vi "Flush.vi"(8 "error in (no error)":errorcluster, 9 "Single / Multivalve?":bool, 10 "Channel":u32, 11 "LINX Resource":T1={"IO"=enum."Remote", "Interface"=enum."Serial", "LINX Device Config"={"Interface"=enum."Serial", "COM Port"="COM13", "TCP Configuration"={"IP Address"="", "Port"=0}, "Device Family"=1, "Device ID"=1, "Device Name"="myRIO-1900", "TCP Ref"=refnum, "Channels"={"DI"=[0, 1, 2, 3, 4, 5, 6, 7, 8, 9, 10, 11, 12, 13, 14, 15, 16, 17, 18, 19, 20, 21, 22, 23, 24, 25, 26, 27, 28, 29, 30, 31, 32, 33, 34, 35, 36, 37, 38, 39, 40, 41, 42, 43, 44, 45, 46], "DO"=[0, 1, 2, 3, 4, 5, 6, 7, 8, 9, 10, 11, 12, 13, 14, 15, 16, 17, 18, 19, 20, 21, 22, 23, 24, 25, 26, 27, 28, 29, 30, 31, 32, 33, 34, 35, 36, 37, 38, 39, 40, 41, 42, 43, 44, 45, 46], "AI"=[0, 1, 2, 3, 4, 5, 6, 7, 8, 9, 10, 11], "AO"=[], "PWM"=[3, 5, 6, 9, 10], "QE"=[], "UART"=[0, 1], "I2C 2"=[0], "SPI"=[0], "CAN"=[], "Servo"=[], "AI Ref (V)"=0.0, "AI Resolution (Bits)"=0, "AO Ref (V)"=0.0, "AO Resolution (Bits)"=0}}}) -> (0 "error out":errorcluster, 3 "LINX Resource out":T1)   [LabVIEW 2018]
uses:
  <vilib>/MakerHub/LINX/Private/Type Defs/LINX Ref.ctl
  <vilib>/MakerHub/LINX/Private/Type Defs/Platform.ctl
  <vilib>/MakerHub/LINX/Private/Type Defs/Interface.ctl
  <vilib>/MakerHub/LINX/Private/Device/Type Defs/LINX Device Config.ctl
  <vilib>/MakerHub/LINX/Private/Device/Type Defs/TCP Config.ctl
  <vilib>/MakerHub/LINX/Private/Device/Type Defs/Channels.ctl
  <vilib>/MakerHub/LINX/Public/Peripherals/Digital/Digital Write N Chans.vi
  <vilib>/MakerHub/LINX/Private/Local IO/LinxDigitalWrite.vi
  <vilib>/MakerHub/LINX/Public/Utilities/Check Channel.vi
  <vilib>/MakerHub/LINX/Private/Utilties/Generate Error.vi
  <vilib>/MakerHub/LINX/LMH-LINX.lvlib
  <vilib>/MakerHub/LINX/Private/Device/Device.lvlib
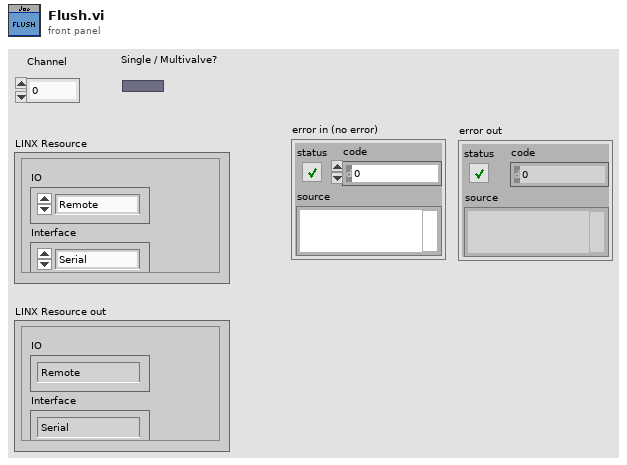
[diagram p1: front panel]
types:
  T1 = typedef "LMH-LINX.lvlib/LINX Ref.ctl" = cluster{"IO":T2, "Interface":T3, "LINX Device Config":T4}
  T2 = typedef "LMH-LINX.lvlib/Platform.ctl" = enum16{"Remote", "Local"}
  T3 = typedef "LMH-LINX.lvlib/Interface.ctl" = enum16{"Serial", "TCP"}
  T4 = typedef "LMH-LINX.lvlib/Device.lvlib/LINX Device Config.ctl" = cluster{"Interface":T3, "COM Port":refnum<visa-resource-name>, "TCP Configuration":T5, "Device Family":u8, "Device ID":u8, "Device Name":string, "TCP Ref":refnum<k5>, "Channels":T6}
  T5 = typedef "LMH-LINX.lvlib/Device.lvlib/TCP Config.ctl" = cluster{"IP Address":string, "Port":u16}
  T6 = typedef "LMH-LINX.lvlib/Channels.ctl" = cluster{"DI":u8[], "DO":u8[], "AI":u8[], "AO":u8[], "PWM":u8[], "QE":u8[], "UART":u8[], "I2C 2":u8[], "SPI":u8[], "CAN":u8[], "Servo":u8[], "AI Ref (V)":dbl, "AI Resolution (Bits)":u8, "AO Ref (V)":dbl, "AO Resolution (Bits)":u8}
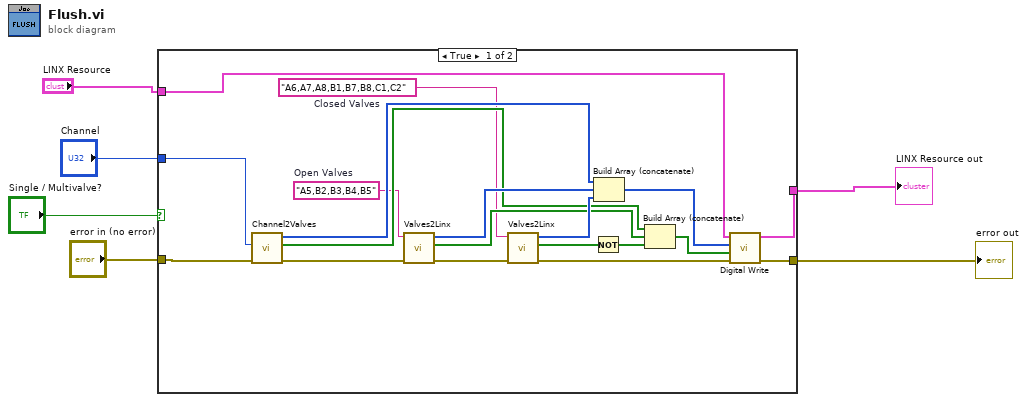
[diagram p0: block diagram]
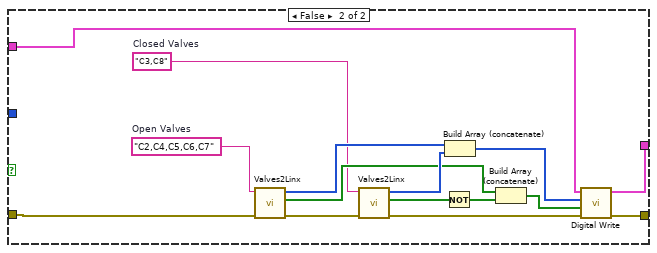
[diagram p2: hidden frame]
diagram:
  n1 = case shown="True" "Single / Multivalve?" {
    tunnel: "error in (no error)" -> [w25 w26]
    tunnel: [w24 w40] -> w5
    tunnel: [w23 w39] -> w4
    tunnel: "Channel" -> [w8 _]
    tunnel: "LINX Resource" -> [w7 w27]
    frame True {
      w9 = "A6,A7,A8,B1,B7,B8,C1,C2"  # Closed Valves
      w10 = "A5,B2,B3,B4,B5"  # Open Valves
      n2 = call "Channel2Valves.vi"("Channel"=w8, "error in (no error)"=w25) -> ("Valve Nums"=w15:i32[], "Valve State"=w14:bool[], "error out"=w13:errorcluster)  [unwired: 6 in]
      n3 = call "Valves2Linx.vi"("error in (no error)"=w13, "Valve (A1-C8),\n comma separated"=w10) -> ("error out"=w17:errorcluster, "Array"=w19:bool[], "Array 2"=w20:i32[])  [unwired: 7 in]
      n4 = call "Valves2Linx.vi"("error in (no error)"=w17, "Valve (A1-C8),\n comma separated"=w9) -> ("error out"=w12:errorcluster, "Array"=w22:bool[], "Array 2"=w21:i32[])  [unwired: 7 in]
      n5 = Not(x=w22) -> (.not. x?=w18:bool[])
      n6 = Build Array (concatenate)(w15, w20, w21) -> (w16:i32[])
      n7 = Build Array (concatenate)(w14, w19, w18) -> (w11:bool[])
      n8 = call-poly <vilib>:"Digital Write.vi"("Error In"=w12, "Values"=w11, "DO Channels"=w16, "LINX Resource"=w7) -> ("Error Out"=w24:errorcluster, "LINX Resource"=w23:T1)  [unwired: 6 in]
    }
    frame False {
      w28 = "C3,C8"  # Closed Valves
      w29 = "C2,C4,C5,C6,C7"  # Open Valves
      n9 = call "Valves2Linx.vi"("error in (no error)"=w26, "Valve (A1-C8),\n comma separated"=w29) -> ("error out"=w33:errorcluster, "Array"=w35:bool[], "Array 2"=w36:i32[])  [unwired: 7 in]
      n10 = call "Valves2Linx.vi"("error in (no error)"=w33, "Valve (A1-C8),\n comma separated"=w28) -> ("error out"=w31:errorcluster, "Array"=w38:bool[], "Array 2"=w37:i32[])  [unwired: 7 in]
      n11 = Not(x=w38) -> (.not. x?=w34:bool[])
      n12 = Build Array (concatenate)(w36, w37) -> (w32:i32[])
      n13 = Build Array (concatenate)(w35, w34) -> (w30:bool[])
      n14 = call-poly <vilib>:"Digital Write.vi"("Error In"=w31, "Values"=w30, "DO Channels"=w32, "LINX Resource"=w27) -> ("Error Out"=w40:errorcluster, "LINX Resource"=w39:T1)  [unwired: 6 in]
    }
  }
  "error out" <- w5
  "LINX Resource out" <- w4
